vi "Tone Glide LUT Demo.vi"() -> ()   [LabVIEW 2015]
uses:
  Utility VIs/Math VIs/LinSpace (x0-dx-npts).vi
panel:
  out "x-y":dbl
  out "Waveform Graph":dbl[](graph)
  in  "F2 (Hz)":dbl=200.0
  in  "F1 (Hz)":dbl=100.0
  in  "Table Res (Hz)":dbl=0.25
  in  "Npts":i32=5000
  in  "Fs":dbl=50000.0
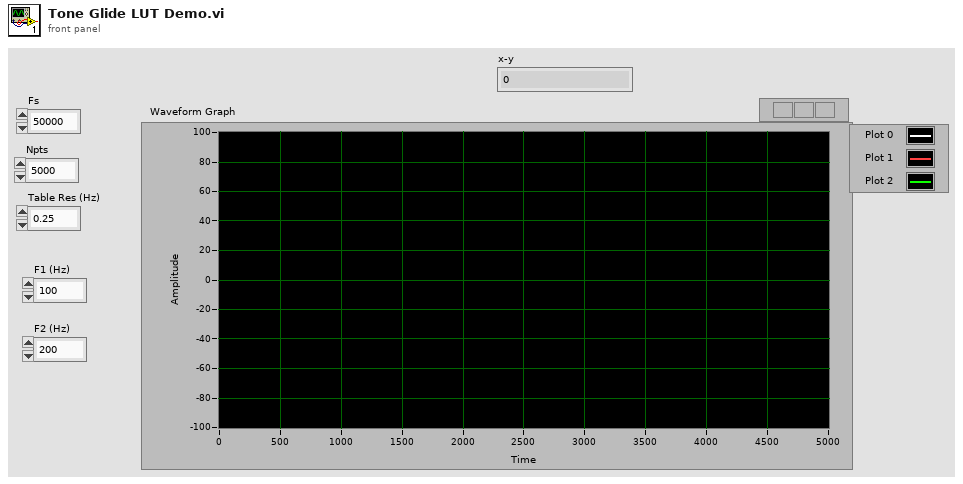
[diagram p1: front panel]
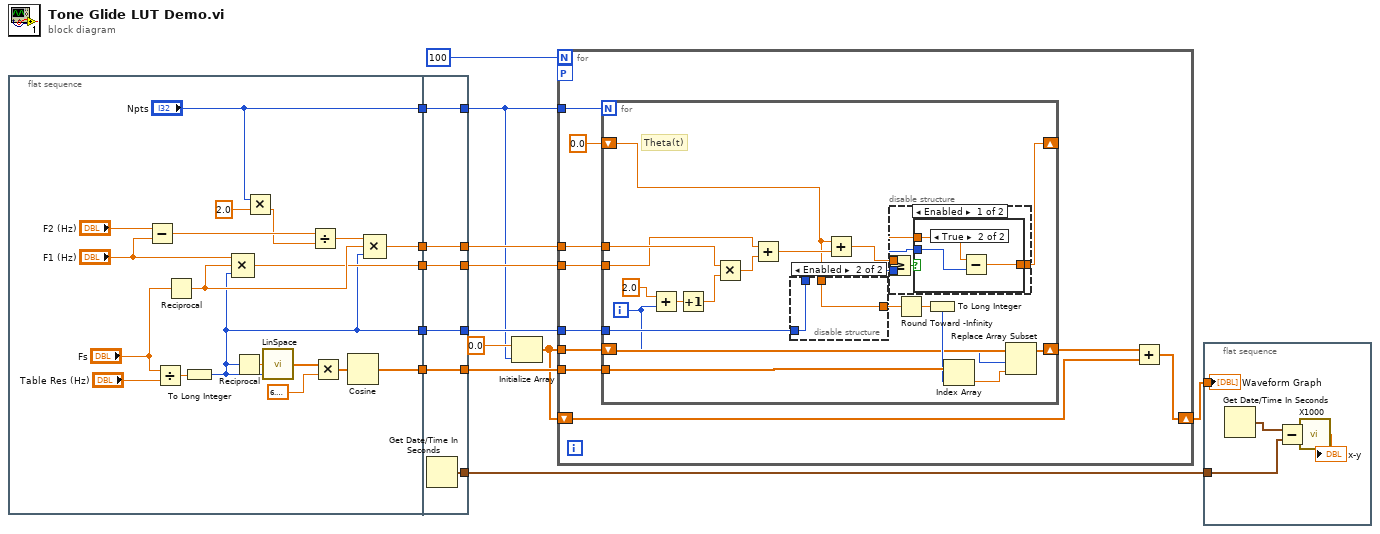
[diagram p0: block diagram]
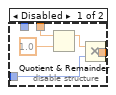
[diagram p4: hidden frame]
diagram:
  n1 = flat-sequence {
    tunnel: [w23] -> w9
    tunnel: [w21] -> w8
    tunnel: [w20] -> w7
    tunnel: [w16] -> w6
    tunnel: ["Npts"] -> w5
    tunnel: [w36] -> w3
    tunnel: [w37] -> w12
    tunnel: [w38] -> w13
    tunnel: [w39] -> w14
    tunnel: [w40] -> w15
    tunnel: w9 -> [w40]
    tunnel: w8 -> [w39]
    tunnel: w7 -> [w38]
    tunnel: w6 -> [w37]
    tunnel: w5 -> [w36]
    tunnel: [w35] -> w4
    frame #0 {
      n2 = Subtract(x="F2 (Hz)", y="F1 (Hz)") -> (x-y=w29:dbl)
      n3 = Divide(x="Fs", y="Table Res (Hz)") -> (x/y=w34:dbl)
      n4 = Reciprocal(x="Fs") -> (1/x=w22:dbl)
      n5 = To Long Integer(number=w34) -> (32bit integer=w16:i32)
      n6 = Compound Arithmetic op=MULTIPLY("F1 (Hz)", w22, w16) -> (w21:dbl)
      n7 = Reciprocal(x=w16) -> (1/x=w33:dbl)
      n8 = Multiply(x="Npts", y=2.0) -> (x*y=w19:dbl)
      n9 = call-poly "LinSpace.vi"("npts"=w16, "dx"=w33) -> ("Array"=w26:dbl[])  [unwired: 2 in, 1 out]
      n10 = Divide(x=w29, y=w19) -> (x/y=w24:dbl)
      n11 = Multiply(x=w26, y=6.283185307179586) -> (x*y=w31:dbl[])
      n12 = Cosine(x=w31) -> (cos(x)=w20:dbl[])
      n13 = Compound Arithmetic op=MULTIPLY(w24, w22, w16) -> (w23:dbl)
    }
    frame #1 {
      n14 = Get Date/Time In Seconds() -> (seconds since 1Jan1904=w35:timestamp)
    }
  }
  n15 = Initialize Array(0.0 ("element"), w3) -> (w2:dbl[])
  n16 = for {
    N: 100 -> [_]
    tunnel: w15 -> [w49]
    tunnel: w14 -> [w48]
    tunnel: w13 -> [w47]
    tunnel: w12 -> [w46]
    tunnel: w3 -> [w45]
    tunnel: w2 -> [w44]
    shift-right: [w41] -> w1
    shift-left: w2 -> [w42]
    workers-P: _ -> [_]
    n17 = for {
      N: w45 -> [_]
      shift-right: [w51] -> _
      shift-left: 0.0 -> [w54]
      tunnel: w49 -> [w63]
      tunnel: w48 -> [w62]
      tunnel: w47 -> [w65]
      tunnel: w46 -> [w61]
      shift-right: [w60] -> w43
      shift-left: w44 -> [w59]
      i -> [w58]
      # "Theta(t)"
      n18 = Add(x=2.0, y=w58) -> (x+y=w68:dbl)
      n19 = Increment(x=w68) -> (x+1=w67:dbl)
      n20 = Multiply(x=w63, y=w67) -> (x*y=w66:dbl)
      n21 = Add(x=w62, y=w66) -> (x+y=w70:dbl)
      n22 = disable-structure shown="Enabled" {
        disable-tunnel: w54 -> [w84 w86]
        disable-tunnel: w61 -> [w83 w85]
        disable-tunnel: [w82 w86] -> w55
        disable-tunnel: [_ w85] -> w53
        frame Disabled {
          n23 = Quotient & Remainder(x=w84, y=1.0) -> (x-y*floor(x/y)=w81:dbl)  [unwired: 1 out]
          n24 = Multiply(x=w81, y=w83) -> (x*y=w82:dbl)
        }
        frame Enabled {
        }
      }
      n25 = Add(x=w54, y=w70) -> (x+y=w52:dbl)
      n26 = disable-structure shown="Enabled" {
        disable-tunnel: w53 -> [w73 _]
        disable-tunnel: w52 -> [w72 w79]
        disable-tunnel: [w71 w79] -> w51
        frame Enabled {
          n27 = Greater Or Equal?(x=w72, y=w73) -> (x >= y?=w74:bool)
          n28 = case shown="True" w74 {
            tunnel: w72 -> [w75 w77]
            tunnel: w73 -> [_ w78]
            tunnel: [w75 w76] -> w71
            frame False {
            }
            frame True {
              n29 = Subtract(x=w77, y=w78) -> (x-y=w76:dbl)
            }
          }
        }
        frame Disabled {
        }
      }
      n30 = Round Toward -Infinity(1:w55) -> (0:w56:dbl)
      n31 = To Long Integer(number=w56) -> (32bit integer=w64:i32)
      n32 = Index Array(array=w65, index=w64) -> (element=w57:dbl)
      n33 = Replace Array Subset(array=w59, new element=w57, index=w58) -> (w60:dbl[])
    }
    n34 = Add(x=w43, y=w42) -> (x+y=w41:dbl[])
  }
  n35 = flat-sequence {
    tunnel: w1 -> [w91]
    tunnel: w4 -> [w89]
    frame #0 {
      n36 = Get Date/Time In Seconds() -> (seconds since 1Jan1904=w90:timestamp)
      n37 = Subtract(x=w90, y=w89) -> (x-y=w88:dbl)
      n38 = call "X1000.vi"("X"=w88) -> ("X/1000"=→"x-y":dbl)
      "Waveform Graph" <- w91
    }
  }
